vi "myRIO_BRig_RT_dataLC_init.vi"() -> (3 "output_dataLC":u16[](array[numeric]))   [LabVIEW 2014]
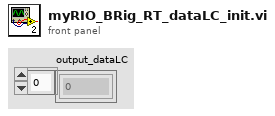
[diagram p1: front panel]
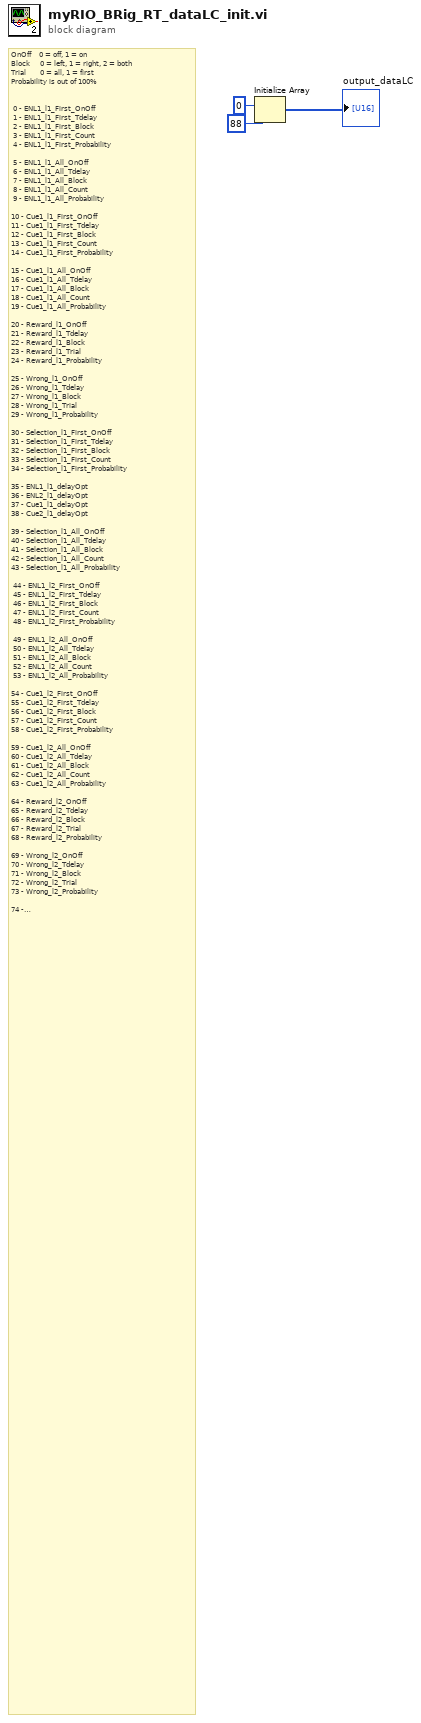
[diagram p0: block diagram]
diagram:
  # "OnOff    0 = off, 1 = on\nBlock     0 = left, 1 = right, 2 = both\nTrial       0 = all, 1 = first\nProbability is out of 100%\n\n\n 0 - ENL1_l1_First_OnOff\n 1 - ENL1_l1_First_Tdelay\n 2 - ENL1_l1_First_Block\n 3 - ENL1_l1_First_Count\n 4 - ENL1_l1_First_Probability\n\n 5 - ENL1_l1_All_OnOff\n 6 - ENL1_l1_All_Tdelay\n 7 - ENL1_l1_All_Block\n 8 - ENL1_l1_All_Count\n 9 - ENL1_l1_All_Probability\n\n10 - Cue1_l1_First_OnOff\n11 - Cue1_l1_First_Tdelay\n12 - Cue1_l1_First_Block\n13 - Cue1_l1_First_Count\n14 - Cue1_l1_First_Probability\n\n15 - Cue1_l1_All_OnOff\n16 - Cue1_l1_All_Tdelay\n17 - Cue1_l1_All_Block\n18 - Cue1_l1_All_Count\n19 - Cue1_l1_All_Probability\n\n20 - Reward_l1_OnOff\n21 - Reward_l1_Tdelay\n22 - Reward_l1_Block\n23 - Reward_l1_Trial\n24 - Reward_l1_Probability\n\n25 - Wrong_l1_OnOff\n26 - Wrong_l1_Tdelay\n27 - Wrong_l1_Block\n28 - Wrong_l1_Trial\n29 - Wrong_l1_Probability\n\n30 - Selection_l1_First_OnOff\n31 - Selection_l1_First_Tdelay\n32 - Selection_l1_First_Block\n33 - Selection_l1_First_Count\n34 - Selection_l1_First_Probability\n\n35 - ENL1_l1_delayOpt\n36 - ENL2_l1_delayOpt\n37 - Cue1_l1_delayOpt\n38 - Cue2_l1_delayOpt\n\n39 - Selection_l1_All_OnOff\n40 - Selection_l1_All_Tdelay\n41 - Selection_l1_All_Block\n42 - Selection_l1_All_Count\n43 - Selection_l1_All_Probability\n\n 44 - ENL1_l2_First_OnOff\n 45 - ENL1_l2_First_Tdelay\n 46 - ENL1_l2_First_Block\n 47 - ENL1_l2_First_Count\n 48 - ENL1_l2_First_Probability\n\n 49 - ENL1_l2_All_OnOff\n 50 - ENL1_l2_All_Tdelay\n 51 - ENL1_l2_All_Block\n 52 - ENL1_l2_All_Count\n 53 - ENL1_l2_All_Probability\n\n54 - Cue1_l2_First_OnOff\n55 - Cue1_l2_First_Tdelay\n56 - Cue1_l2_First_Block\n57 - Cue1_l2_First_Count\n58 - Cue1_l2_First_Probability\n\n59 - Cue1_l2_All_OnOff\n60 - Cue1_l2_All_Tdelay\n61 - Cue1_l2_All_Block\n62 - Cue1_l2_All_Count\n63 - Cue1_l2_All_Probability\n\n64 - Reward_l2_OnOff\n65 - Reward_l2_Tdelay\n66 - Reward_l2_Block\n67 - Reward_l2_Trial\n68 - Reward_l2_Probability\n\n69 - Wrong_l2_OnOff\n70 - Wrong_l2_Tdelay\n71 - Wrong_l2_Block\n72 - Wrong_l2_Trial\n73 - Wrong_l2_Probability\n\n74 - Selection_l2_First_OnOff\n75 - Selection_l2_First_Tdelay\n76 - Selection_l2_First_Block\n77 - Selection_l2_First_Count\n78 - Selection_l2_First_Probability\n\n79 - ENL1_l2_First_delayOpt\n80 - ENL1_l2_All_delayOpt\n81 - Cue1_l2_First_delayOpt\n82 - Cue1_l2_All_delayOpt\n\n83 - Selection_l2_All_OnOff\n84 - Selection_l2_All_Tdelay\n85 - Selection_l2_All_Block\n86 - Selection_l2_All_Count\n87 - Selection_l2_All_Probability"
  n1 = Initialize Array(u16 0 ("element"), 88 ("dimension size")) -> (→"output_dataLC":u16[])
